vi "hw1-2 topVI.vi"() -> ()   [LabVIEW 2014]
panel:
  in  "stop":bool
  out "Waveform Chart":cluster{dbl, dbl, dbl}(graph)
  out "Tie Rate":dbl
  out "Player1 Win Rate 2":dbl
  out "Player1 Win Rate":dbl
  out "Plyer2 avg. dice number":dbl
  out "Plyer1 avg. dice number":dbl
  out "Player2-5":u8
  out "Player2-4":u8
  out "Player2-3":u8
  out "Player2-2":u8
  out "Player2-1":u8
  out "Player1- 5":u8
  out "Player1- 4":u8
  out "Player1- 3":u8
  out "Player1- 2":u8
  out "Player1-1":u8
  out "Result":string
  out "Player1 Dice":u8
  out "Player2 Dice":u8
  out "Dice rolling instr.":string
  out "Player2 finish":bool
  out "Player1 finish":bool
  in  "Player2 roll":bool
  in  "Player1 roll":bool
  # "Steps for each round:\n1. One Player push the OK button to roll the dice first\n2. Another Player push the other OK button to roll the dice\n3. \"Player1 Dice\" and \"Player2 Dice\" will show the dice rolling result for about 0.5 seconds\n4. The result will be push into the \"dice number history stack\" (Player1-1,1-2,.....,Player2-1,2-2,...)\n5. Simultaneously, the \"Win Rate\", \"Tie Rate\", \"avg. dice number\", \"Result String\", \"Waveform\" will be calculated and shown"
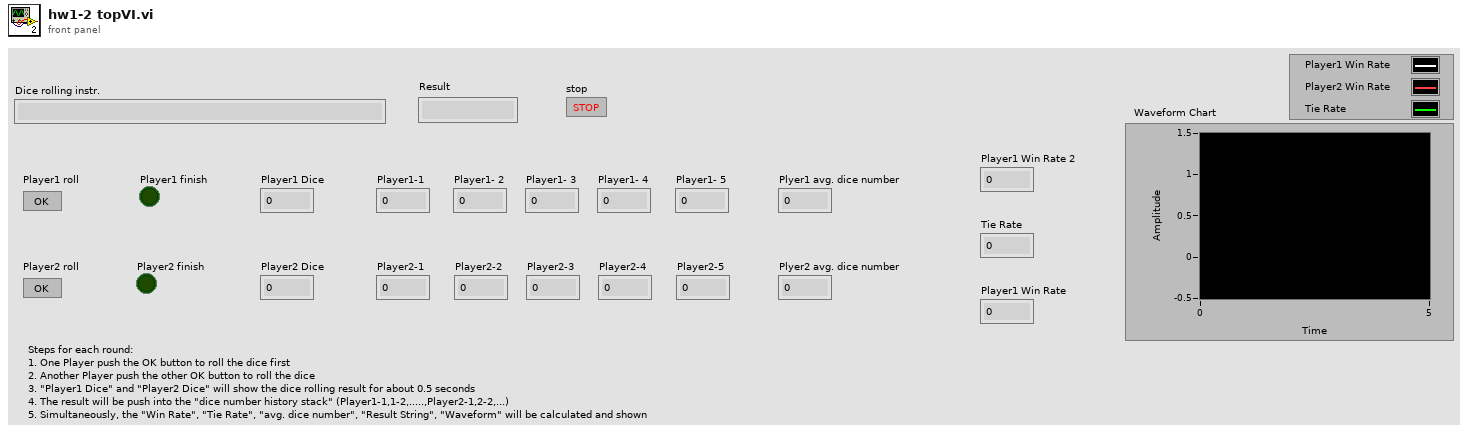
[diagram p1: front panel]
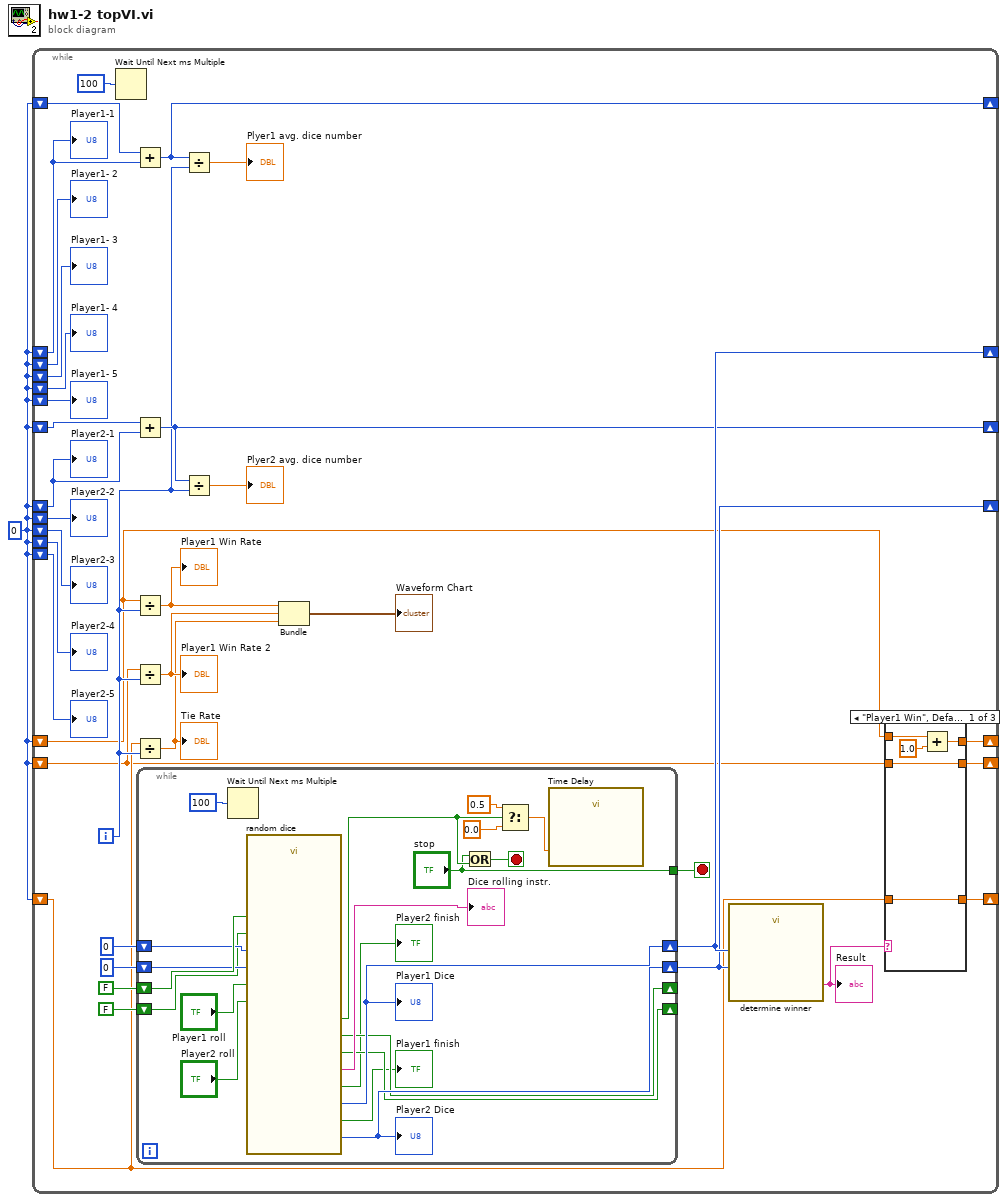
[diagram p0: block diagram]
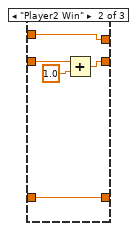
[diagram p2: hidden frame]
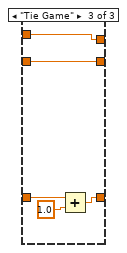
[diagram p3: hidden frame]
diagram:
  w1 = u8 0
  n1 = while {
    shift-right: [w32] -> _
    shift-left: w1 -> [w17]
    shift-right: [w31] -> _
    shift-left: w1 -> [w15]
    shift-left: w1 -> [w29]
    shift-left: w1 -> [w28]
    shift-left: w1 -> [w27]
    shift-left: w1 -> [w26]
    shift-left: w1 -> [w30]
    shift-left: w1 -> [w23]
    shift-left: w1 -> [w24]
    shift-left: w1 -> [w25]
    shift-right: [w19] -> _
    shift-left: w1 -> [w18]
    shift-right: [w20] -> _
    shift-left: w1 -> [w16]
    shift-right: [w10] -> _
    shift-left: w1 -> [w8]
    shift-right: [w11] -> _
    shift-left: w1 -> [w7]
    shift-right: [w12] -> _
    shift-left: w1 -> [w9]
    i -> [w13]
    stop <- w2 stop-if-true
    n2 = Wait Until Next ms Multiple(millisecond multiple=u32 100) -> ()  [unwired: 1 out]
    n3 = Add(x=w18, y=w17) -> (x+y=w19:u8)
    n4 = Add(x=w16, y=w15) -> (x+y=w20:u8)
    n5 = Divide(x=w8, y=w13) -> (x/y=w6:dbl)
    "Player1 Win Rate" <- w6
    n6 = Divide(x=w7, y=w13) -> (x/y=w5:dbl)
    "Player1 Win Rate 2" <- w5
    n7 = Divide(x=w9, y=w13) -> (x/y=w4:dbl)
    "Tie Rate" <- w4
    n8 = while {
      shift-right: [w61] -> _
      shift-left: FALSE -> [w71]
      shift-right: [w67] -> w32
      shift-left: u8 0 -> [w70]
      shift-right: [w62] -> _
      shift-left: FALSE -> [w68]
      shift-right: [w66] -> w31
      shift-left: u8 0 -> [w69]
      tunnel: ["stop"] -> w2
      stop <- w53 stop-if-true
      n9 = Wait Until Next ms Multiple(millisecond multiple=u32 100) -> ()  [unwired: 1 out]
      n10 = call "random dice.vi"("Player1 roll"="Player1 roll", "dice1 state"=w70, "button1 state"=w71, "Player2 roll"="Player2 roll", "button2 state"=w68, "dice2 state"=w69) -> ("Player1 Finish"=→"Player1 finish":bool, "button1 next_state"=w61:bool, "Player1 Dice"=w67:u8, "Player2 Dice"=w66:u8, "Dice rolling instr."=→"Dice rolling instr.":string, "Player2 Finish"=→"Player2 finish":bool, "button2 next_state"=w62:bool, "both finished"=w55:bool)  [unwired: 2 in]
      "Player2 Dice" <- w66
      "Player1 Dice" <- w67
      n11 = Or(x="stop", y=w55) -> (x .or. y?=w53:bool)
      n12 = Select(t=0.5, s=w55, f=0.0) -> (s? t:f=w58:dbl)
      n13 = call "Time Delay"("Delay Time (s)"=w58) -> ()  [unwired: 10 in, 1 out]
    }
    n14 = Divide(x=w19, y=w13) -> (x/y=→"Plyer1 avg. dice number":dbl)
    n15 = Divide(x=w20, y=w13) -> (x/y=→"Plyer2 avg. dice number":dbl)
    n16 = Bundle(w6, w5, w4) -> (→"Waveform Chart":cluster{dbl, dbl, dbl})  [unwired: 1 in]
    n17 = call "determine winner.vi"("Player2"=w31, "Player1"=w32) -> ("Result"=w14:string)  [unwired: 9 in]
    "Result" <- w14
    n18 = case shown="\"Player1 Win\", Default" w14 {
      tunnel: w8 -> [w41 w44 w48]
      tunnel: w7 -> [w39 w46 w49]
      tunnel: w9 -> [w38 w43 w51]
      tunnel: [w38 w43 w50] -> w12
      tunnel: [w39 w45 w49] -> w11
      tunnel: [w40 w44 w48] -> w10
      frame "Player1 Win", Default {
        n19 = Add(x=w41, y=1.0) -> (x+y=w40:dbl)
      }
      frame "Player2 Win" {
        n20 = Add(x=w46, y=1.0) -> (x+y=w45:dbl)
      }
      frame "Tie Game" {
        n21 = Add(x=w51, y=1.0) -> (x+y=w50:dbl)
      }
    }
    "Player1-1" <- w17
    "Player1- 2" <- w29
    "Player1- 3" <- w28
    "Player1- 4" <- w27
    "Player1- 5" <- w26
    "Player2-1" <- w15
    "Player2-2" <- w30
    "Player2-3" <- w23
    "Player2-4" <- w24
    "Player2-5" <- w25
  }
